vi "UR3_model_parse.vi"(10 "Link info":string, 11 "Name":string) -> (1 "Good point?":bool, 2 "Info":T1, 3 "name out":string)   [LabVIEW 2024]
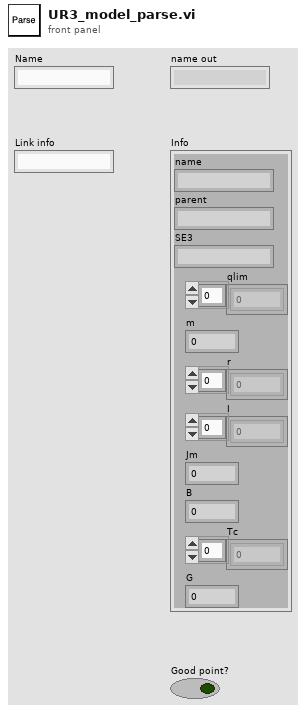
[diagram p1: front panel]
types:
  T1 = cluster{"name":string, "parent":string, "SE3":string, "qlim":dbl[], "m":dbl, "r":dbl[], "I":dbl[], "Jm":dbl, "B":dbl, "Tc":dbl[], "G":dbl}
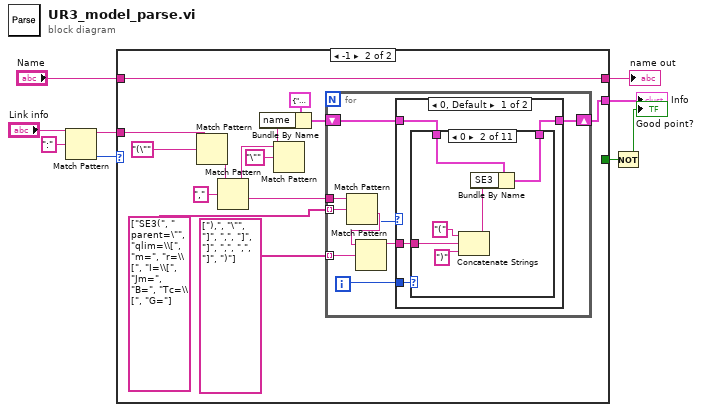
[diagram p0: block diagram]
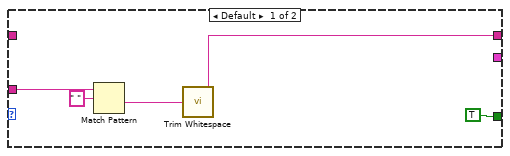
[diagram p2: hidden frame]
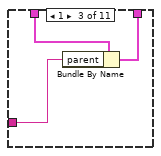
[diagram p4: hidden frame]
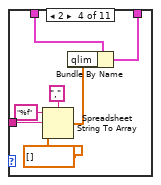
[diagram p5: hidden frame]
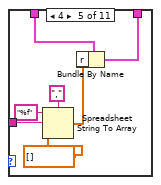
[diagram p6: hidden frame]
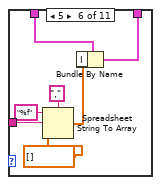
[diagram p7: hidden frame]
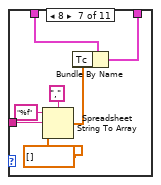
[diagram p8: hidden frame]
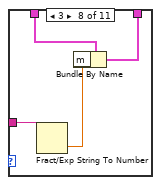
[diagram p9: hidden frame]
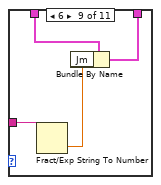
[diagram p10: hidden frame]
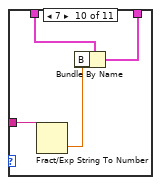
[diagram p11: hidden frame]
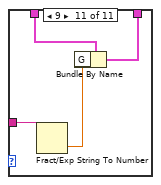
[diagram p12: hidden frame]
diagram:
  n1 = Match Pattern(string="Link info", regular expression=":") -> (before substring=w3:string, offset past match=w9:i32)  [unwired: 1 in, 2 out]
  n2 = case shown="-1" w9 {
    tunnel: w3 -> [w13 w27]
    tunnel: [w11 w21] -> w5
    tunnel: "Name" -> [_ w21]
    tunnel: [_ w20] -> w6
    tunnel: [TRUE _] -> w7
    frame Default {
      n3 = Match Pattern(string=w13, regular expression=" ") -> (after substring=w12:string)  [unwired: 1 in, 3 out]
      n4 = call <vilib>:"Trim Whitespace.vi"("string"=w12) -> ("trimmed string"=w11:string)  [unwired: 1 in]
    }
    frame -1 {
      n5 = Match Pattern(string=w27, regular expression="(\"") -> (after substring=w25:string)  [unwired: 1 in, 3 out]
      n6 = Match Pattern(string=w25, regular expression=",") -> (before substring=w16:string, after substring=w24:string)  [unwired: 1 in, 2 out]
      n7 = Match Pattern(string=w16, regular expression="\"") -> (before substring=w15:string)  [unwired: 1 in, 3 out]
      n8 = Bundle By Name(cluster=T1 {"name"="", "parent"="", "SE3"="", "qlim"=[], "m"=0.0, "r"=[], "I"=[], "Jm"=0.0, "B"=0.0, "Tc"=[], "G"=0.0}, "name"=w15) -> (w19:T1)
      n9 = for {
        tunnel: w24 -> [w36]
        tunnel: string[] ["SE3(", " parent=\"", "qlim=\\[", "m=", "r=\\[", "I=\\[", "Jm=", "B=", "Tc=\\[", "G="] -> [w35] mode=indexing
        tunnel: string[] ["),", "\"", "]", ",", "]", "]", ",", ",", "]", ")"] -> [w34] mode=indexing
        shift-right: [w31] -> w20
        shift-left: w19 -> [w29]
        i -> [w32]
        n10 = Match Pattern(string=w36, regular expression=w35) -> (after substring=w37:string, offset past match=w33:i32)  [unwired: 1 in, 2 out]
        n11 = Match Pattern(string=w37, regular expression=w34) -> (before substring=w30:string)  [unwired: 1 in, 3 out]
        n12 = case shown="0, Default" w33 {
          tunnel: w32 -> [w41 _]
          tunnel: [w39 w96] -> w31
          tunnel: w29 -> [w40 w96]
          tunnel: w30 -> [w38 _]
          frame 0, Default {
            n13 = case shown="0" w41 {
              tunnel: w40 -> [w42 w48 w51 w58 w65 w72 w79 w83 w87 w91 w95]
              tunnel: [w42 w47 w50 w57 w64 w71 w78 w82 w86 w90 w94] -> w39
              tunnel: w38 -> [_ w46 w49 w56 w63 w70 w77 w81 w85 w89 w93]
              frame Default {
              }
              frame 0 {
                n14 = Concatenate Strings("(" ("regular expression"), w46, ")" ("regular expression")) -> (w45:string)
                n15 = Bundle By Name(cluster=w48, "SE3"=w45) -> (w47:T1)
              }
              frame 1 {
                n16 = Bundle By Name(cluster=w51, "parent"=w49) -> (w50:T1)
              }
              frame 2 {
                n17 = Spreadsheet String To Array(delimiter (Tab)=",", format string="%f", spreadsheet string=w56, array type (2D Dbl)=dbl[] [] ("qlim")) -> (array=w52:dbl[])
                n18 = Bundle By Name(cluster=w58, "qlim"=w52) -> (w57:T1)
              }
              frame 4 {
                n19 = Spreadsheet String To Array(delimiter (Tab)=",", format string="%f", spreadsheet string=w63, array type (2D Dbl)=dbl[] [] ("qlim")) -> (array=w59:dbl[])
                n20 = Bundle By Name(cluster=w65, "r"=w59) -> (w64:T1)
              }
              frame 5 {
                n21 = Spreadsheet String To Array(delimiter (Tab)=",", format string="%f", spreadsheet string=w70, array type (2D Dbl)=dbl[] [] ("qlim")) -> (array=w66:dbl[])
                n22 = Bundle By Name(cluster=w72, "I"=w66) -> (w71:T1)
              }
              frame 8 {
                n23 = Spreadsheet String To Array(delimiter (Tab)=",", format string="%f", spreadsheet string=w77, array type (2D Dbl)=dbl[] [] ("qlim")) -> (array=w73:dbl[])
                n24 = Bundle By Name(cluster=w79, "Tc"=w73) -> (w78:T1)
              }
              frame 3 {
                n25 = Fract/Exp String To Number(string=w81) -> (number=w80:dbl)  [unwired: 3 in, 1 out]
                n26 = Bundle By Name(cluster=w83, "m"=w80) -> (w82:T1)
              }
              frame 6 {
                n27 = Fract/Exp String To Number(string=w85) -> (number=w84:dbl)  [unwired: 3 in, 1 out]
                n28 = Bundle By Name(cluster=w87, "Jm"=w84) -> (w86:T1)
              }
              frame 7 {
                n29 = Fract/Exp String To Number(string=w89) -> (number=w88:dbl)  [unwired: 3 in, 1 out]
                n30 = Bundle By Name(cluster=w91, "B"=w88) -> (w90:T1)
              }
              frame 9 {
                n31 = Fract/Exp String To Number(string=w93) -> (number=w92:dbl)  [unwired: 3 in, 1 out]
                n32 = Bundle By Name(cluster=w95, "G"=w92) -> (w94:T1)
              }
            }
          }
          frame -1 {
          }
        }
      }
    }
  }
  "Info" <- w6
  "name out" <- w5
  n33 = Not(x=w7) -> (.not. x?=→"Good point?":bool)
